vi "queue.vi"() -> ()   [LabVIEW 2012]
panel:
  in  "string":string
  out "element":string
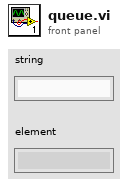
[diagram p1: front panel]
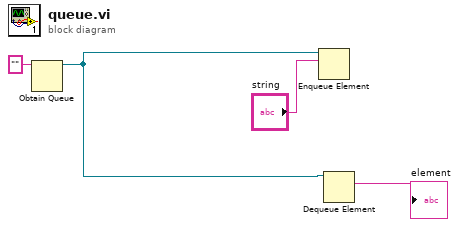
[diagram p0: block diagram]
diagram:
  n1 = Obtain Queue(name (unnamed)="") -> (queue out=w4:refnum<queue>)  [unwired: 4 in, 2 out]
  n2 = Enqueue Element(queue=w4, element="string") -> ()  [unwired: 2 in, 3 out]
  n3 = Dequeue Element(queue=w4) -> (element=→"element":string)  [unwired: 2 in, 3 out]
